vi "WPI_MotorControlEnable.vi"(8 "error in (no error)":errorcluster, 10 "Encoder Initial Position":dbl, 11 "CAN MotorDevRef":T1={"DeviceStatus"={"status"=FALSE, "code"=0, "source"=""}, "Type"=enum."PWM", "PWM"={"PWM Channel"=enum."Invalid", "DeadBand"={"Name"="", "maxPositivePwm"=0, "minPositivePwm"=0, "centerPwm"=0, "maxNegativePwm"=0, "minNegativePwm"=0, "angularRange"=0}}, "CAN"={"Device Number"=0, "SetOutput VI Ref"=variant(refnum<vi> refnum), "GetOutput VI Ref"=variant(refnum<vi> refnum), "Enable VI Ref"=variant(refnum<vi> refnum), "Disable VI Ref"=variant(refnum<vi> refnum), "Data"=variant}, "Invert"=FALSE, "DIO PWM"={"PWM \"Enable\" Channel"=enum."Invalid", "DIOChannel"=enum."Invalid", "PWM Rate"=0.0}}) -> (0 "error out":errorcluster, 3 "CAN MotorDevRef":T1={"DeviceStatus"={"status"=FALSE, "code"=0, "source"=""}, "Type"=enum."PWM", "PWM"={"PWM Channel"=enum."Invalid", "DeadBand"={"Name"="", "maxPositivePwm"=0, "minPositivePwm"=0, "centerPwm"=0, "maxNegativePwm"=0, "minNegativePwm"=0, "angularRange"=0}}, "CAN"={"Device Number"=0, "SetOutput VI Ref"=variant(refnum<vi> refnum), "GetOutput VI Ref"=variant(refnum<vi> refnum), "Enable VI Ref"=variant(refnum<vi> refnum), "Disable VI Ref"=variant(refnum<vi> refnum), "Data"=variant}, "Invert"=FALSE, "DIO PWM"={"PWM \"Enable\" Channel"=enum."Invalid", "DIOChannel"=enum."Invalid", "PWM Rate"=0.0}})   [LabVIEW 2025]
doc: "Enable the closed loop controller in the <B>Control Mode</B> that was specified in <B>Open</B> on a CAN Jaguar. You must also call this VI after calling the <B>Change Mode</B> VI to start the closed loop controller.\n\nThis software is licensed. Open the labview\\readme\\WPI Robotics Library Open Source License.txt file for more information."
uses:
  <vilib>/Rock Robotics/WPI/MotorControl/WPI_MotorControlDeviceRef.ctl
  <vilib>/Rock Robotics/WPI/MotorControl/WPI_MotorControlType.ctl
  <vilib>/Rock Robotics/SystemInterfaces/DIO/FPGA_DIOPWMChannel.ctl
  <vilib>/Rock Robotics/WPI/PWM/WPI_PWMDeadband.ctl
  <vilib>/Rock Robotics/SystemInterfaces/DIO/FPGA_DIOChannel.ctl
  <vilib>/Rock Robotics/WPI/MotorControl/WPI_MotorControlEnableRefType.ctl
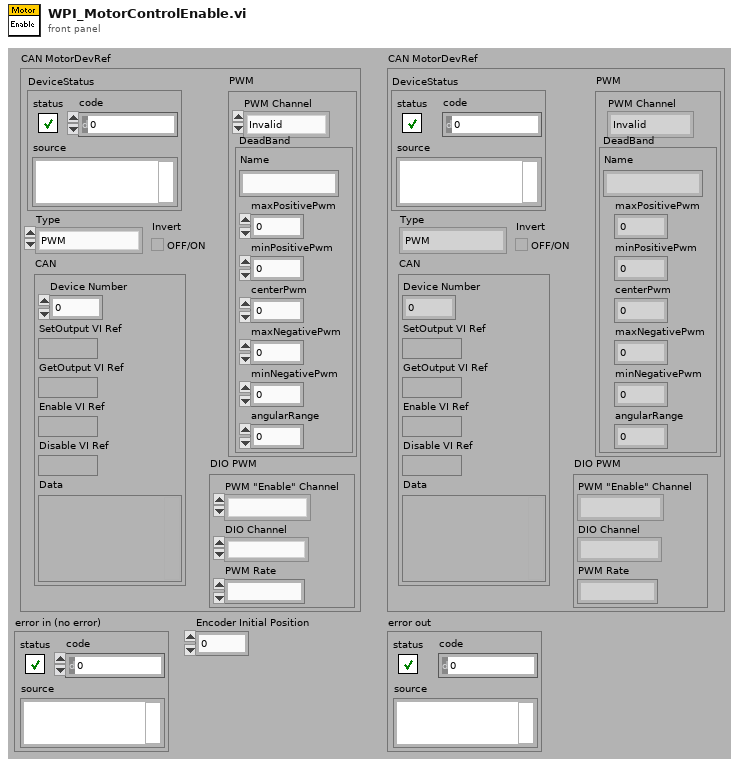
[diagram p1: front panel]
types:
  T1 = typedef "WPI_MotorControlDeviceRef.ctl" = cluster{"DeviceStatus":errorcluster, "Type":T2, "PWM":cluster{"PWM Channel":T3, "DeadBand":T4}, "CAN":cluster{"Device Number":u8, "SetOutput VI Ref":variant, "GetOutput VI Ref":variant, "Enable VI Ref":variant, "Disable VI Ref":variant, "Data":variant}, "Invert":bool, "DIO PWM":cluster{"PWM \"Enable\" Channel":T3, "DIOChannel":T5, "PWM Rate":dbl}}
  T2 = typedef "WPI_MotorControlType.ctl" = enum16{"PWM", "CAN", "DIO PWM"}
  T3 = typedef "FPGA_DIOPWMChannel.ctl" = enum8{"PWM 0", "PWM 1", "PWM 2", "PWM 3", "PWM 4", "PWM 5", "PWM 6", "PWM 7", "PWM 8", "PWM 9", "PWM MXP 0", "PWM MXP 1", "PWM MXP 2", "PWM MXP 3", "PWM MXP 4", "PWM MXP 5", "PWM MXP 6", "PWM MXP 7", "PWM MXP 8", "PWM MXP 9", "Invalid"}
  T4 = typedef "WPI_PWMDeadband.ctl" = cluster{"Name":string, "maxPositivePwm":i32, "minPositivePwm":i32, "centerPwm":i32, "maxNegativePwm":i32, "minNegativePwm":i32, "angularRange":u16}
  T5 = typedef "FPGA_DIOChannel.ctl" = enum8{"DIO 0", "DIO 1", "DIO 2", "DIO 3", "DIO 4", "DIO 5", "DIO 6", "DIO 7", "DIO 8", "DIO 9", "DIO MXP 0", "DIO MXP 1", "DIO MXP 2", "DIO MXP 3", "DIO MXP 4", "DIO MXP 5", "DIO MXP 6", "DIO MXP 7", "DIO MXP 8", "DIO MXP 9", "DIO MXP 10", "DIO MXP 11", "DIO MXP 12", "DIO MXP 13", "DIO MXP 14", "DIO MXP 15", "SPI Port CS1", "SPI Port CS2", "SPI Port CS3", "SPI Port MISO", "SPI Port MOSI", "Invalid"}
  T6 = typedef "WPI_MotorControlEnableRefType.ctl" = refnum<vi>
  T7 = typedef "WPI_PWMDeviceRef.ctl" = cluster{"DeviceStatus":errorcluster, "PWM Channel":T3}
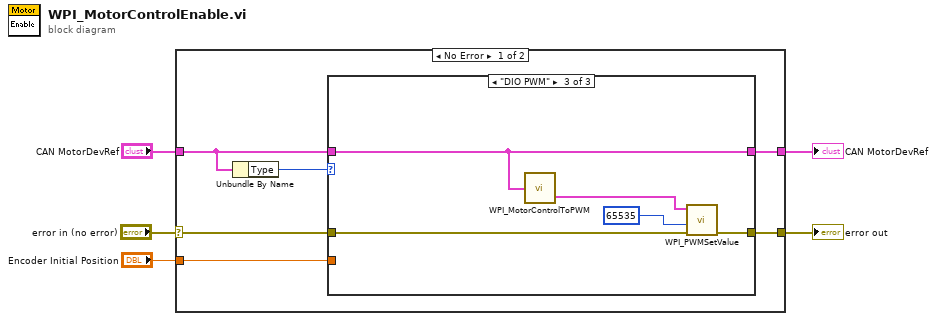
[diagram p0: block diagram]
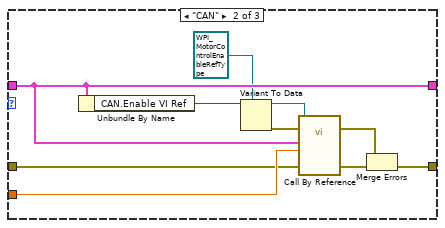
[diagram p3: hidden frame]
diagram:
  n1 = case shown="No Error" "error in (no error)" {
    selector: "error in (no error)" -> [w6 w29]
    tunnel: "CAN MotorDevRef" -> [w10 w28]
    tunnel: [w8 w28] -> w4
    tunnel: [w9 w29] -> w3
    tunnel: "Encoder Initial Position" -> [w11 _]
    frame No Error {
      n2 = Unbundle By Name(w10) -> ("Type"=w7:T2)
      n3 = case shown="\"DIO PWM\"" w7 {
        tunnel: w11 -> [_ w22 _]
        tunnel: w10 -> [w12 w19 w24]
        tunnel: [_ w15 w25] -> w9
        tunnel: [w12 w19 w24] -> w8
        tunnel: w6 -> [_ w21 w26]
        frame "PWM" {
        }
        frame "CAN" {
          n4 = Unbundle By Name(w19) -> ("CAN.Enable VI Ref"=w20:variant)
          n5 = Variant To Data(type=T6 refnum ("MotorControlSetOutput"), Variant=w20) -> (data=w17:T6, error out=w18:errorcluster)  [unwired: 1 in]
          n6 = call-by-ref "?"(reference=w17, error in=w18, 8:"error in (no error)"=w21, "Encoder Initial Position"=w22, "CAN MotorDevRef"=w19) -> (error out=w14:errorcluster, 0:"error out"=w16:errorcluster)  [unwired: 7 in, 2 out]
          n7 = Merge Errors(w14, w16) -> (w15:errorcluster)
        }
        frame "DIO PWM" {
          n8 = call <vilib>:"WPI_MotorControlToPWM.vi"("MotorControlDeviceRef"=w24) -> ("PWMDeviceRef"=w23:T7)  [unwired: 1 out]
          n9 = call <vilib>:"WPI_PWMSetValue.vi"("error in (no error)"=w26, "Value"=u16 65535, "PWMDeviceRef"=w23) -> ("error out"=w25:errorcluster)  [unwired: 7 in, 1 out]
        }
      }
    }
    frame Error {
    }
  }
  "error out" <- w3
  "CAN MotorDevRef" <- w4
